vi "Get All Projects.vi"(8 "error in":errorcluster, 11 "Project Selection":string) -> (0 "error out":errorcluster, 1 "Application":refnum<vi>, 2 "Project Name":string, 3 "My Computer Target":refnum<vi>, 5 "Project":refnum<vi>)   [LabVIEW 2019, in "Panther Dashboard.lvlib"]
uses:
  Panther Dashboard.lvlib
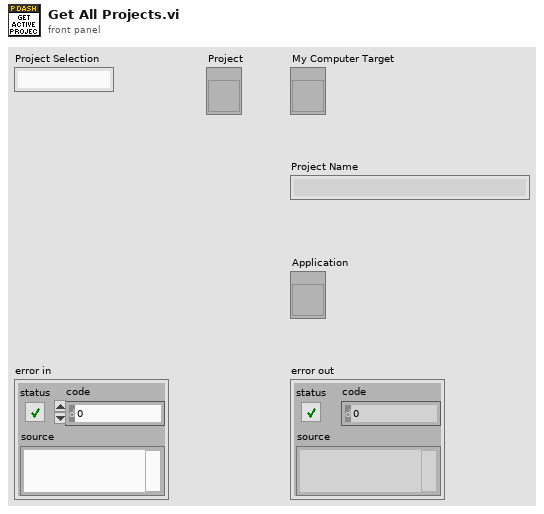
[diagram p1: front panel]
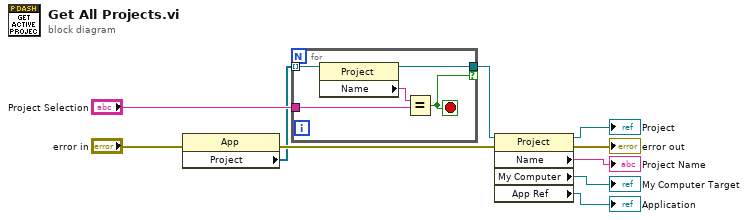
[diagram p0: block diagram]
diagram:
  n1 = property class="App"(error in="error in") -> (error out=w8:errorcluster, "Project"=w1:refnum<vi>[])  [unwired: 1 in, 1 out]
  n2 = for {
    tunnel: w1 -> [w15] mode=indexing
    tunnel: [w13] -> w3 if=w12
    tunnel: "Project Selection" -> [w11]
    stop <- w12 stop-if-true
    n3 = property class="Project"(reference=w15) -> (reference out=w13:refnum<vi>, "Name"=w14:string)  [unwired: 1 in, 1 out]
    n4 = Equal?(x=w14, y=w11) -> (x = y?=w12:bool)
  }
  n5 = property class="Project"(reference=w3, error in=w8) -> (reference out=→"Project":refnum<vi>, error out=→"error out":errorcluster, "Name"=→"Project Name":string, "My Computer"=→"My Computer Target":refnum<vi>, "App Ref"=→"Application":refnum<vi>)
